vi "SetWaitForAnyVI_popup.vi"(0 "Input Line Command":string, 3 "error in (no error)":errorcluster, 4 "Control Name":string, 7 "Value":string) -> (8 "error out":errorcluster, 9 "Cancel":bool, 10 "Output Line Command":string)   [LabVIEW 2019]
panel:
  in  "Remote computer IP":string
  in  "platform":u16(ring) items=["Mac", "PC"]
  in  "Timeout":string
  in  "Condition":string(combo)
  in  "Target VI":string
  in  "Cancel button":bool
  in  "OK Button":bool
  # "(empty: local host)"
  # "(number only)"
  # "(larger, smaller or close to (within 1%))"
  # "For remote connection:\nGo to the VI server setting (Tools-> Options) of the server (remote) computer.\n(1) TCP/IP checked.\n(2) Verify and use the port #\n(3) Add host IP (this computer) in the Machin Access list."
  # "min"
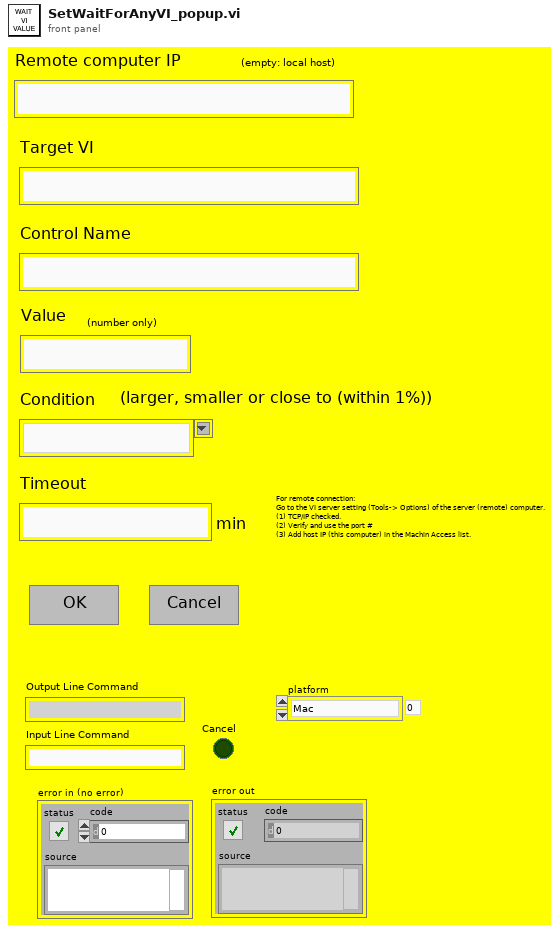
[diagram p1: front panel]
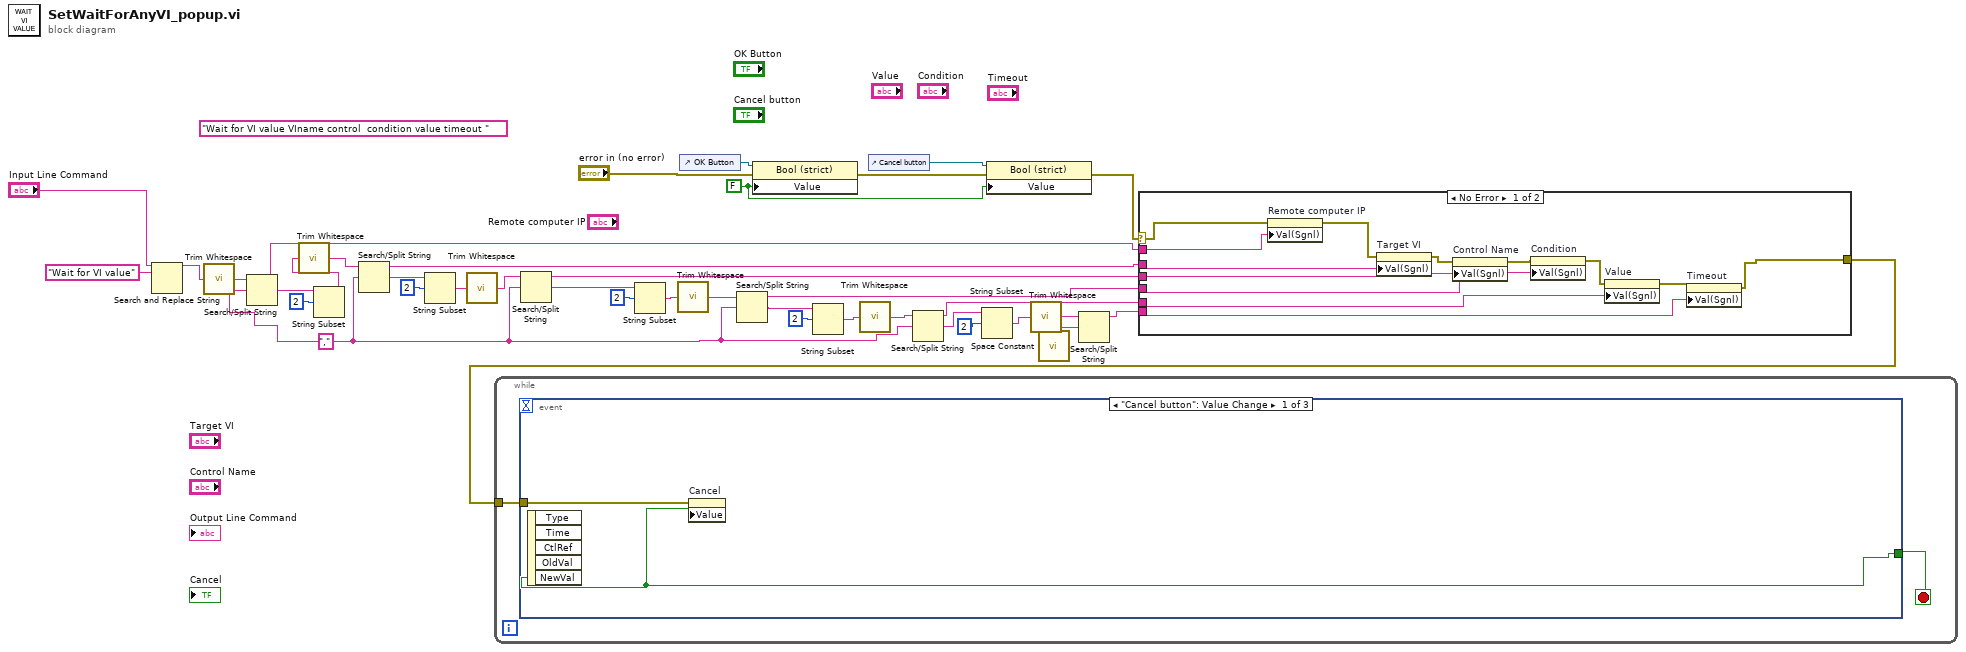
[diagram p0: block diagram]
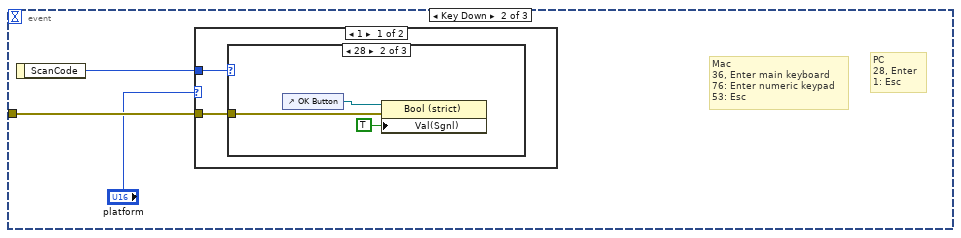
[diagram p2: hidden frame]
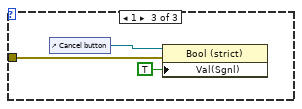
[diagram p4: hidden frame]
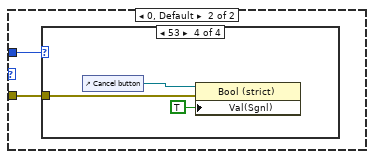
[diagram p5: hidden frame]
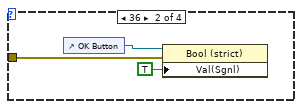
[diagram p7: hidden frame]
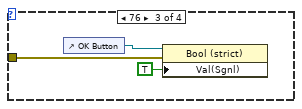
[diagram p8: hidden frame]
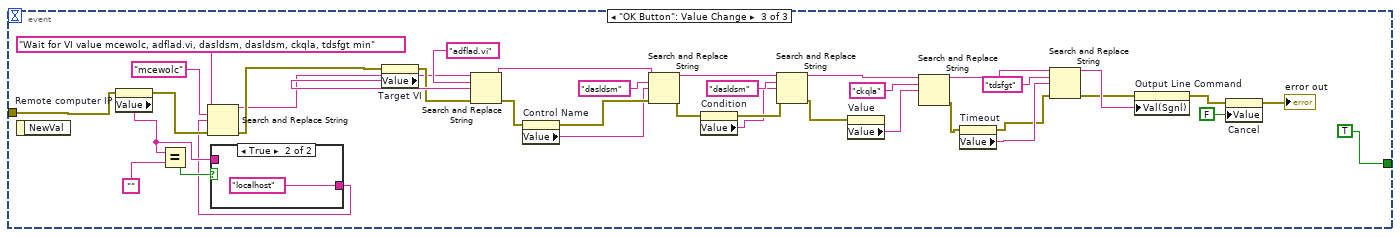
[diagram p9: hidden frame]
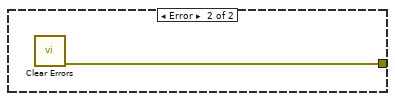
[diagram p11: hidden frame]
diagram:
  (unwired) "Wait for VI value VIname control  condition value timeout " ("format string")
  w5 = "," ("search string/char (-)")
  w39 = FALSE
  n1 = Search and Replace String(input string="Input Line Command", search string="Wait for VI value") -> (result string=w6:string)  [unwired: 6 in, 3 out]
  n2 = call <vilib>:"Trim Whitespace.vi"("string"=w6) -> ("trimmed string"=w7:string)  [unwired: 1 in]
  n3 = Search/Split String(string=w7, search string/char (-)=w5) -> (substring before match=w1:string, match + rest of string=w3:string)  [unwired: 1 in, 1 out]
  n4 = String Subset(string=w3, offset (0)=2) -> (substring=w2:string)  [unwired: 1 in]
  n5 = call <vilib>:"Trim Whitespace.vi"("string"=w2) -> ("trimmed string"=w30:string)  [unwired: 1 in]
  n6 = Search/Split String(string=w30, search string/char (-)=w5) -> (substring before match=w20:string, match + rest of string=w28:string)  [unwired: 1 in, 1 out]
  n7 = String Subset(string=w28, offset (0)=2) -> (substring=w27:string)  [unwired: 1 in]
  n8 = call <vilib>:"Trim Whitespace.vi"("string"=w27) -> ("trimmed string"=w32:string)  [unwired: 1 in]
  n9 = Search/Split String(string=w32, search string/char (-)=w5) -> (substring before match=w19:string, match + rest of string=w25:string)  [unwired: 1 in, 1 out]
  n10 = String Subset(string=w25, offset (0)=2) -> (substring=w24:string)  [unwired: 1 in]
  n11 = call <vilib>:"Trim Whitespace.vi"("string"=w24) -> ("trimmed string"=w31:string)  [unwired: 1 in]
  n12 = control-ref of="OK Button"() -> (w38:refnum<vi>)
  n13 = Search/Split String(string=w31, search string/char (-)=w5) -> (substring before match=w18:string, match + rest of string=w14:string)  [unwired: 1 in, 1 out]
  n14 = property on="Property Node" class="Bool (strict)"(reference=w38, error in="error in (no error)", "Value"=w39) -> (error out=w35:errorcluster)  [unwired: 1 out]
  n15 = String Subset(string=w14, offset (0)=2) -> (substring=w15:string)  [unwired: 1 in]
  n16 = call <vilib>:"Trim Whitespace.vi"("string"=w15) -> ("trimmed string"=w13:string)  [unwired: 1 in]
  n17 = control-ref of="Cancel button"() -> (w37:refnum<vi>)
  n18 = Search/Split String(string=w13, search string/char (-)=w5) -> (substring before match=w11:string, match + rest of string=w12:string)  [unwired: 1 in, 1 out]
  n19 = String Subset(string=w12, offset (0)=2) -> (substring=w22:string)  [unwired: 1 in]
  n20 = property on="Property Node" class="Bool (strict)"(reference=w37, error in=w35, "Value"=w39) -> (error out=w17:errorcluster)  [unwired: 1 out]
  n21 = call <vilib>:"Trim Whitespace.vi"("string"=w22) -> ("trimmed string"=w10:string)  [unwired: 1 in]
  n22 = call <vilib>:"Space Constant.vi"() -> ("String"=w9:string)
  n23 = Search/Split String(string=w10, search string/char (-)=w9) -> (substring before match=w8:string)  [unwired: 1 in, 2 out]
  n24 = case shown="No Error" w17 {
    selector: w17 -> [w42 _]
    tunnel: [w49 w53] -> w34
    tunnel: w20 -> [w51 _]
    tunnel: w19 -> [w50 _]
    tunnel: w18 -> [w47 _]
    tunnel: w8 -> [w48 _]
    tunnel: w11 -> [w46 _]
    tunnel: w1 -> [w40 _]
    frame No Error {
      n25 = property on="Remote computer IP" class="Str"(error in=w42, "Val(Sgnl)"=w40) -> (error out=w41:errorcluster)  [unwired: 1 in, 1 out]
      n26 = property on="Target VI" class="Str"(error in=w41, "Val(Sgnl)"=w51) -> (error out=w52:errorcluster)  [unwired: 1 in, 1 out]
      n27 = property on="Control Name" class="Str"(error in=w52, "Val(Sgnl)"=w50) -> (error out=w45:errorcluster)  [unwired: 1 in, 1 out]
      n28 = property on="Condition" class="CmbBox"(error in=w45, "Val(Sgnl)"=w47) -> (error out=w44:errorcluster)  [unwired: 1 in, 1 out]
      n29 = property on="Value" class="Str"(error in=w44, "Val(Sgnl)"=w46) -> (error out=w43:errorcluster)  [unwired: 1 in, 1 out]
      n30 = property on="Timeout" class="Str"(error in=w43, "Val(Sgnl)"=w48) -> (error out=w49:errorcluster)  [unwired: 1 in, 1 out]
    }
    frame Error {
      n31 = call <vilib>:"Clear Errors.vi"() -> ("error out"=w53:errorcluster)  [unwired: 6 in, 1 out]
    }
  }
  n32 = while {
    tunnel: w34 -> [w55]
    stop <- w54 stop-if-true
    n33 = event shown="[0] \"Cancel button\": Value Change" {
      selector: _ -> [_ _ _]
      dyn-events: _ -> [_ _ _]
      timeout: _ -> [_ _ _]
      tunnel: w55 -> [w57 w59 w89]
      tunnel: [w56 _ TRUE] -> w54
      event "Cancel button": Value Change {
        n34 = event-data() -> ("NewVal"=w56:bool)  [unwired: 1 in, 4 out]
        n35 = property on="Cancel" class="Bool (strict)"(error in=w57, "Value"=w56) -> ()  [unwired: 1 in, 2 out]
      }
      event Key Down {
        # "PC\n28, Enter \n1: Esc"
        # "Mac\n36, Enter main keyboard\n76: Enter numeric keypad\n53: Esc"
        n36 = event-data() -> ("ScanCode"=w60:i16)  [unwired: 1 in]
        n37 = case shown="1" "platform" {
          tunnel: w60 -> [w62 w70]
          tunnel: w59 -> [w61 w69]
          frame 1 {
            n38 = case shown="28" w62 {
              tunnel: w61 -> [_ w65 w67]
              frame Default {
              }
              frame 28 {
                n39 = control-ref of="OK Button"() -> (w63:refnum<vi>)
                n40 = property on="Property Node" class="Bool (strict)"(reference=w63, error in=w65, "Val(Sgnl)"=TRUE ("Value (Signaling)")) -> ()  [unwired: 2 out]
              }
              frame 1 {
                n41 = control-ref of="Cancel button"() -> (w66:refnum<vi>)
                n42 = property on="Property Node" class="Bool (strict)"(reference=w66, error in=w67, "Val(Sgnl)"=TRUE ("Value (Signaling)")) -> ()  [unwired: 2 out]
              }
            }
          }
          frame 0, Default {
            n43 = case shown="53" w70 {
              tunnel: w69 -> [_ w73 w76 w78]
              frame Default {
              }
              frame 36 {
                n44 = control-ref of="OK Button"() -> (w71:refnum<vi>)
                n45 = property on="Property Node" class="Bool (strict)"(reference=w71, error in=w73, "Val(Sgnl)"=TRUE ("Value (Signaling)")) -> ()  [unwired: 2 out]
              }
              frame 76 {
                n46 = control-ref of="OK Button"() -> (w74:refnum<vi>)
                n47 = property on="Property Node" class="Bool (strict)"(reference=w74, error in=w76, "Val(Sgnl)"=TRUE ("Value (Signaling)")) -> ()  [unwired: 2 out]
              }
              frame 53 {
                n48 = control-ref of="Cancel button"() -> (w77:refnum<vi>)
                n49 = property on="Property Node" class="Bool (strict)"(reference=w77, error in=w78, "Val(Sgnl)"=TRUE ("Value (Signaling)")) -> ()  [unwired: 2 out]
              }
            }
          }
        }
      }
      event "OK Button": Value Change {
        n50 = event-data() -> ()  [unwired: 1 in, 1 out]
        n51 = property on="Remote computer IP" class="Str"(error in=w89) -> (error out=w87:errorcluster, "Value"=w81:string)  [unwired: 1 in, 1 out]
        n52 = Equal?(x=w81, y="") -> (x = y?=w82:bool)
        n53 = case shown="True" w82 {
          tunnel: [w118 "localhost" ("search string")] -> w80
          tunnel: w81 -> [w118 _]
          frame False {
          }
          frame True {
          }
        }
        n54 = Search and Replace String(input string="Wait for VI value mcewolc, adflad.vi, dasldsm, dasldsm, ckqla, tdsfgt min" ("format string"), search string="mcewolc", replace string=w80, error in=w87) -> (result string=w83:string, error out=w86:errorcluster)  [unwired: 4 in, 2 out]
        n55 = property on="Target VI" class="Str"(error in=w86) -> (error out=w104:errorcluster, "Value"=w105:string)  [unwired: 1 in, 1 out]
        n56 = Search and Replace String(input string=w83, search string="adflad.vi", replace string=w105, error in=w104) -> (result string=w107:string, error out=w103:errorcluster)  [unwired: 4 in, 2 out]
        n57 = property on="Control Name" class="Str"(error in=w103) -> (error out=w111:errorcluster, "Value"=w110:string)  [unwired: 1 in, 1 out]
        n58 = Search and Replace String(input string=w107, search string="dasldsm", replace string=w110, error in=w111) -> (result string=w116:string, error out=w95:errorcluster)  [unwired: 4 in, 2 out]
        n59 = property on="Condition" class="CmbBox"(error in=w95) -> (error out=w94:errorcluster, "Value"=w91:string)  [unwired: 1 in, 1 out]
        n60 = Search and Replace String(input string=w116, search string="dasldsm", replace string=w91, error in=w94) -> (result string=w109:string, error out=w93:errorcluster)  [unwired: 4 in, 2 out]
        n61 = property on="Value" class="Str"(error in=w93) -> ("Value"=w92:string)  [unwired: 1 in, 2 out]
        n62 = Search and Replace String(input string=w109, search string="ckqla", replace string=w92) -> (result string=w101:string, error out=w100:errorcluster)  [unwired: 5 in, 2 out]
        n63 = property on="Timeout" class="Str"(error in=w100) -> (error out=w98:errorcluster, "Value"=w99:string)  [unwired: 1 in, 1 out]
        n64 = Search and Replace String(input string=w101, search string="tdsfgt", replace string=w99, error in=w98) -> (result string=w97:string, error out=w96:errorcluster)  [unwired: 4 in, 2 out]
        n65 = property on="Output Line Command" class="Str"(error in=w96, "Val(Sgnl)"=w97) -> (error out=w114:errorcluster)  [unwired: 1 in, 1 out]
        n66 = property on="Cancel" class="Bool (strict)"(error in=w114, "Value"=FALSE ("Cancel")) -> (error out=→"error out":errorcluster)  [unwired: 1 in, 1 out]
      }
    }
  }
